vi "Utility Decode ID String.vi"(8 "error in (no error)":errorcluster, 10 "*IDN? Response":string, 11 "VISA resource name in":refnum<visa-resource-name>) -> (0 "error out":errorcluster, 2 "Unit Info":T1, 3 "VISA resource name out":refnum<visa-resource-name>)   [LabVIEW 2019, in "Quantum Composers 9000 Series.lvlib"]
doc: "This VI decodes the response from an *IDN? query to return information about the unit It is private in scope."
uses:
  Quantum Composers 9000 Series.lvlib
  Unit Info.ctl
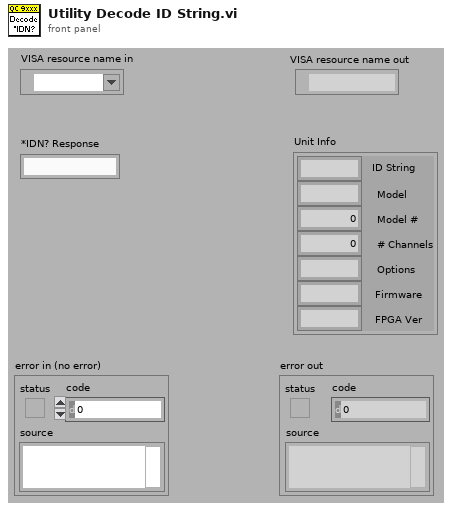
[diagram p1: front panel]
types:
  T1 = typedef "Quantum Composers 9000 Series.lvlib/Unit Info.ctl" = cluster{"ID String":string, "Model":string, "Model #":i32, "# Channels":i32, "Options":string, "Firmware":string, "FPGA Ver":string}
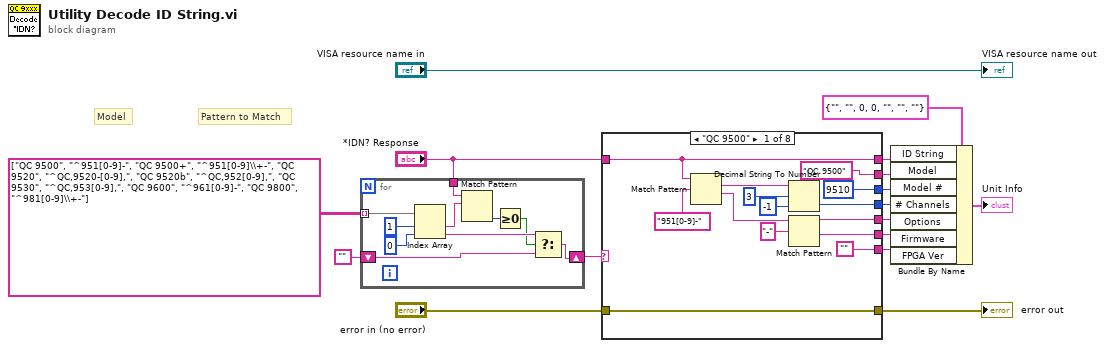
[diagram p0: block diagram]
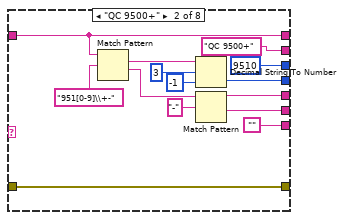
[diagram p2: hidden frame]
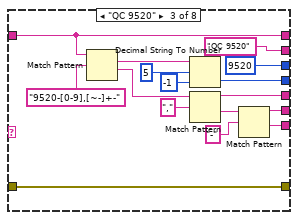
[diagram p3: hidden frame]
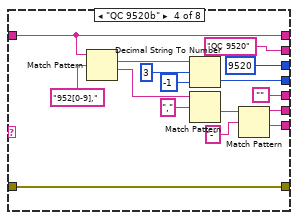
[diagram p4: hidden frame]
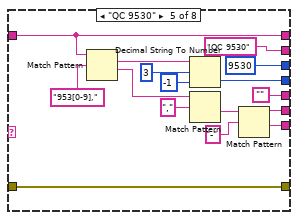
[diagram p5: hidden frame]
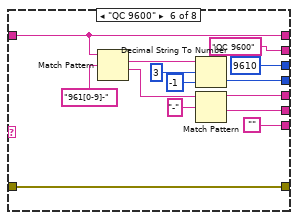
[diagram p6: hidden frame]
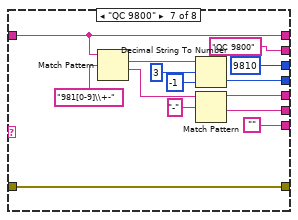
[diagram p7: hidden frame]
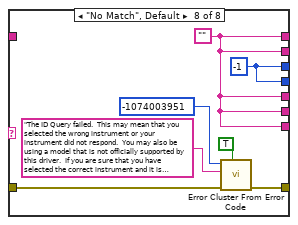
[diagram p8: hidden frame]
diagram:
  # "Pattern to Match"
  # "Model"
  n1 = for {
    tunnel: string[][] [["QC 9500", "^951[0-9]-"], ["QC 9500+", "^951[0-9]\\+-"], ["QC 9520", "^QC,9520-[0-9],"], ["QC 9520b", "^QC,952[0-9],"], ["QC 9530", "^QC,953[0-9],"], ["QC 9600", "^961[0-9]-"], ["QC 9800", "^981[0-9]\\+-"]] ("appended array") -> [w24] mode=indexing
    tunnel: "*IDN? Response" -> [w25]
    shift-right: [w18] -> w6
    shift-left: "" -> [w19]
    n2 = Index Array(array=w24, index #1=1 ("index"), index #2=0 ("index")) -> (element #1=w23:string, element #2=w20:string)
    n3 = Match Pattern(string=w25, regular expression=w23) -> (offset past match=w26:i32)  [unwired: 1 in, 3 out]
    n4 = Greater Or Equal To 0?(x=w26) -> (x >= 0?=w17:bool)
    n5 = Select(t=w20, s=w17, f=w19) -> (s? t:f=w18:string)
  }
  n6 = case shown="\"QC 9500\"" w6 {
    tunnel: "*IDN? Response" -> [w38 w52 w68 w84 w100 w114 w128 _]
    tunnel: [w38 w52 w68 w84 w100 w114 w128 w136] -> w7
    tunnel: ["QC 9500" ("Model") "QC 9500+" ("Model") "QC 9520" ("Model") "QC 9520" ("Model") "QC 9530" ("Model") "QC 9600" ("Model") "QC 9800" ("Model") w136] -> w8
    tunnel: [9510 ("Model #") 9510 ("Model #") 9520 ("Model #") 9520 ("Model #") 9530 ("Model #") 9610 ("Model #") 9810 ("Model #") w137] -> w9
    tunnel: [w35 w49 w65 w81 w97 w111 w125 w137] -> w10
    tunnel: [w31 w45 w63 "" "" w107 w121 w136] -> w11
    tunnel: [w30 w44 w58 w75 w91 w106 w120 w136] -> w12
    tunnel: ["" "" w57 w74 w90 "" "" w136] -> w13
    tunnel: "error in (no error)" -> [w27 w41 w55 w72 w88 w103 w117 w132]
    tunnel: [w27 w41 w55 w72 w88 w103 w117 w131] -> w4
    frame "QC 9500" {
      n7 = Match Pattern(string=w38, regular expression="951[0-9]-") -> (match substring=w34:string, after substring=w32:string)  [unwired: 1 in, 2 out]
      n8 = Decimal String To Number(string=w34, offset=3, default (0L)=-1) -> (number=w35:i32)  [unwired: 1 out]
      n9 = Match Pattern(string=w32, regular expression="-") -> (before substring=w31:string, after substring=w30:string)  [unwired: 1 in, 2 out]
    }
    frame "QC 9500+" {
      n10 = Match Pattern(string=w52, regular expression="951[0-9]\\+-") -> (match substring=w48:string, after substring=w46:string)  [unwired: 1 in, 2 out]
      n11 = Decimal String To Number(string=w48, offset=3, default (0L)=-1) -> (number=w49:i32)  [unwired: 1 out]
      n12 = Match Pattern(string=w46, regular expression="-") -> (before substring=w45:string, after substring=w44:string)  [unwired: 1 in, 2 out]
    }
    frame "QC 9520" {
      n13 = Match Pattern(string=w68, regular expression="9520-[0-9],[~-]+-") -> (match substring=w62:string, after substring=w61:string)  [unwired: 1 in, 2 out]
      n14 = Decimal String To Number(string=w62, offset=5, default (0L)=-1) -> (number=w65:i32)  [unwired: 1 out]
      n15 = Match Pattern(string=w61, regular expression=",") -> (before substring=w63:string, after substring=w59:string)  [unwired: 1 in, 2 out]
      n16 = Match Pattern(string=w59, regular expression="-") -> (before substring=w58:string, after substring=w57:string)  [unwired: 1 in, 2 out]
    }
    frame "QC 9520b" {
      n17 = Match Pattern(string=w84, regular expression="952[0-9],") -> (match substring=w79:string, after substring=w78:string)  [unwired: 1 in, 2 out]
      n18 = Decimal String To Number(string=w79, offset=3, default (0L)=-1) -> (number=w81:i32)  [unwired: 1 out]
      n19 = Match Pattern(string=w78, regular expression=",") -> (after substring=w76:string)  [unwired: 1 in, 3 out]
      n20 = Match Pattern(string=w76, regular expression="-") -> (before substring=w75:string, after substring=w74:string)  [unwired: 1 in, 2 out]
    }
    frame "QC 9530" {
      n21 = Match Pattern(string=w100, regular expression="953[0-9],") -> (match substring=w95:string, after substring=w94:string)  [unwired: 1 in, 2 out]
      n22 = Decimal String To Number(string=w95, offset=3, default (0L)=-1) -> (number=w97:i32)  [unwired: 1 out]
      n23 = Match Pattern(string=w94, regular expression=",") -> (after substring=w92:string)  [unwired: 1 in, 3 out]
      n24 = Match Pattern(string=w92, regular expression="-") -> (before substring=w91:string, after substring=w90:string)  [unwired: 1 in, 2 out]
    }
    frame "QC 9600" {
      n25 = Match Pattern(string=w114, regular expression="961[0-9]-") -> (match substring=w110:string, after substring=w108:string)  [unwired: 1 in, 2 out]
      n26 = Decimal String To Number(string=w110, offset=3, default (0L)=-1) -> (number=w111:i32)  [unwired: 1 out]
      n27 = Match Pattern(string=w108, regular expression="-") -> (before substring=w107:string, after substring=w106:string)  [unwired: 1 in, 2 out]
    }
    frame "QC 9800" {
      n28 = Match Pattern(string=w128, regular expression="981[0-9]\\+-") -> (match substring=w124:string, after substring=w122:string)  [unwired: 1 in, 2 out]
      n29 = Decimal String To Number(string=w124, offset=3, default (0L)=-1) -> (number=w125:i32)  [unwired: 1 out]
      n30 = Match Pattern(string=w122, regular expression="-") -> (before substring=w121:string, after substring=w120:string)  [unwired: 1 in, 2 out]
    }
    frame "No Match", Default {
      w137 = -1 ("Model #")
      w136 = ""
      n31 = call <vilib>:"Error Cluster From Error Code.vi"("show call chain? (False)"=TRUE, "error in (no error)"=w132, "error message (\"\")"="The ID Query failed.  This may mean that you selected the wrong instrument or your instrument did not respond.  You may also be using a model that is not officially supported by this driver.  If you are sure that you have selected the correct instrument and it is responding, try disabling the ID Query." ("Source (VI Name)"), "error code (0)"=-1074003951 ("Code")) -> ("error out"=w131:errorcluster)  [unwired: 5 in]
    }
  }
  "error out" <- w4
  n32 = Bundle By Name(cluster=T1 {"ID String"="", "Model"="", "Model #"=0, "# Channels"=0, "Options"="", "Firmware"="", "FPGA Ver"=""} ("Unit Info"), "ID String"=w7, "Model"=w8, "Model #"=w9, "# Channels"=w10, "Options"=w11, "Firmware"=w12, "FPGA Ver"=w13) -> (→"Unit Info":T1)
  "VISA resource name out" <- "VISA resource name in"
